vi "RT_Thrust_Force_in_DLR_Body_Reference_System(SubVI).vi"(6 "Act_b(i)":dbl[](array[numeric]), 8 "Nzl_S":dbl, 9 "i":i32, 10 "Patm (Pa)":dbl, 11 "Data":dbl[][](array[numeric])) -> (3 "FE_b":dbl[](array[numeric]))   [LabVIEW 2011]
panel:
  out "Fez":dbl
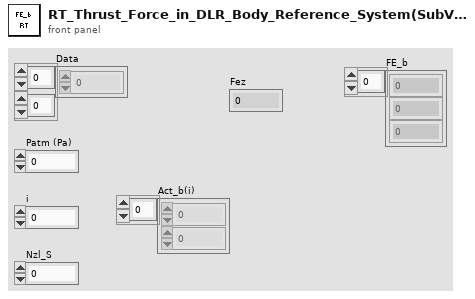
[diagram p1: front panel]
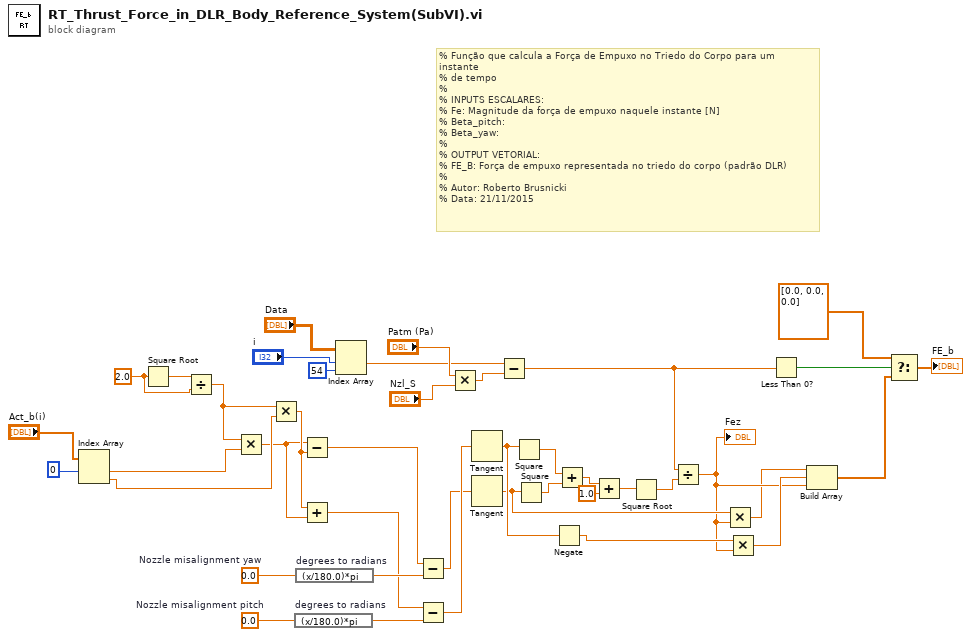
[diagram p0: block diagram]
diagram:
  w11 = 2.0 ("x")
  w14 = 0.0  # Nozzle misalignment pitch
  w13 = 0.0  # Nozzle misalignment yaw
  # "% Função que calcula a Força de Empuxo no Triedo do Corpo para um instante\n% de tempo\n%\n% INPUTS ESCALARES:\n% Fe: Magnitude da força de empuxo naquele instante [N]\n% Beta_pitch: \n% Beta_yaw:\n%\n% OUTPUT VETORIAL:\n% FE_B: Força de empuxo representada no triedo do corpo (padrão DLR)\n%\n% Autor: Roberto Brusnicki\n% Data: 21/11/2015"
  n1 = Index Array(array="Act_b(i)", index #1=0 ("disabled index (col)")) -> (element #1=w10:dbl, element #2=w8:dbl)  [unwired: 1 in]
  n2 = Square Root(x=w11) -> (sqrt(x)=w12:dbl)
  n3 = Divide(x=w12, y=w11) -> (x/y=w9:dbl)
  n4 = Multiply(x=w9, y=w10) -> (x*y=w5:dbl)
  n5 = Multiply(x=w9, y=w8) -> (x*y=w6:dbl)
  n6 = expression code="(x/180.0)*pi" "degrees to radians"(w14) -> (w15:dbl)
  n7 = expression code="(x/180.0)*pi" "degrees to radians"(w13) -> (w16:dbl)
  n8 = Subtract(x=w5, y=w6) -> (x-y=w7:dbl)
  n9 = Add(x=w6, y=w5) -> (x+y=w4:dbl)
  n10 = Index Array(array="Data", index (row)="i", index (col)=54 ("disabled index (col)")) -> (element=w1:dbl)
  n11 = Subtract(x=w7, y=w16) -> (x-y=w2:dbl)
  n12 = Subtract(x=w4, y=w15) -> (x-y=w3:dbl)
  n13 = Multiply(x="Patm (Pa)", y="Nzl_S") -> (x*y=w25:dbl)
  n14 = Tangent(1:w3) -> (0:w36:dbl)
  n15 = Tangent(1:w2) -> (0:w35:dbl)
  n16 = Subtract(x=w1, y=w25) -> (x-y=w19:dbl)
  n17 = Square(x=w36) -> (x^2=w28:dbl)
  n18 = Square(x=w35) -> (x^2=w27:dbl)
  n19 = Negate(x=w36) -> (-x=w37:dbl)
  n20 = Add(x=w28, y=w27) -> (x+y=w29:dbl)
  n21 = Add(x=w29, y=1.0) -> (x+y=w31:dbl)
  n22 = Square Root(x=w31) -> (sqrt(x)=w32:dbl)
  n23 = Divide(x=w19, y=w32) -> (x/y=w34:dbl)
  "Fez" <- w34
  n24 = Multiply(x=w35, y=w34) -> (x*y=w33:dbl)
  n25 = Multiply(x=w37, y=w34) -> (x*y=w38:dbl)
  n26 = Less Than 0?(x=w19) -> (x < 0?=w26:bool)
  n27 = Build Array(w33, w38, w34) -> (w40:dbl[])
  n28 = Select(t=dbl[] [0.0, 0.0, 0.0], s=w26, f=w40) -> (s? t:f=→"FE_b":dbl[])
